vi "acsweep.vi"() -> ()   [LabVIEW 2010]
doc: "I. Description:\nThis example demonstrates how to take a single Measurement (Sample) from an Analog Input Channel.\n\nII. Instructions for Running:\n1. Select the Physical Channel to correspond to where your signal is input on the DAQ device.\n2. Enter the Minimum and Maximum Voltage Ranges\nNote: For better accuracy try to match the Input Ranges to the expected voltage level of the measured signal.\nNote: Use the Gen Voltage Update example to provide a signal on your DAQ device to measure.\n\nIII. Block Diagram Steps:\n1. Create an Analog Input Voltage Channel.\n2. Use the Read VI to Measure 1 Sample from 1 Channel on the Data\nAcquisition Card. Set a timeout so an error is returned if the sample\nis not returned in the specified time limit\n3. Call the Clear Task VI to clear the Task.\n4. Use the popup dialog box to display an error if any.\n\nIV. I/O Connections Overview:\nMake sure your signal input terminal matches the Physical Channel I/O Control."
uses:
  <vilib>/Utility/file.llb/Write To Spreadsheet File (DBL).vi
panel:
  out "Waveform Output":dbl[](graph)
  in  "Physical Channel 2":tag="Dev1/ao0"
  in  "Amplitud":dbl=10.0
  in  "Duracion (s)":dbl=1.0
  in  "stop 2":bool
  out "Waveform Input":dbl[](graph)
  out "Paso #":i32
  in  "Freq Paso":dbl step=0.001 format="%0.3f"
  in  "Freq Hasta":dbl step=0.001 format="%0.3f"
  in  "Freq Desde":dbl step=0.001 format="%0.3f"
  out "Numeric":u32
  in  "Corre":bool
  in  "Maximum Value 2":dbl=10.0 caption="Maximum Value" format="%.2f"
  in  "Minimum Value 2":dbl=-10.0 caption="Minimum Value" format="%0.2f"
  out "In Range?":bool
  in  "stop":bool
  in  "Maximum Value":dbl=10.0 format="%.2f"
  in  "Minimum Value":dbl=-10.0 format="%0.2f"
  in  "Physical Channel":tag="Dev1/ai0"
  # "Channel Parameters"
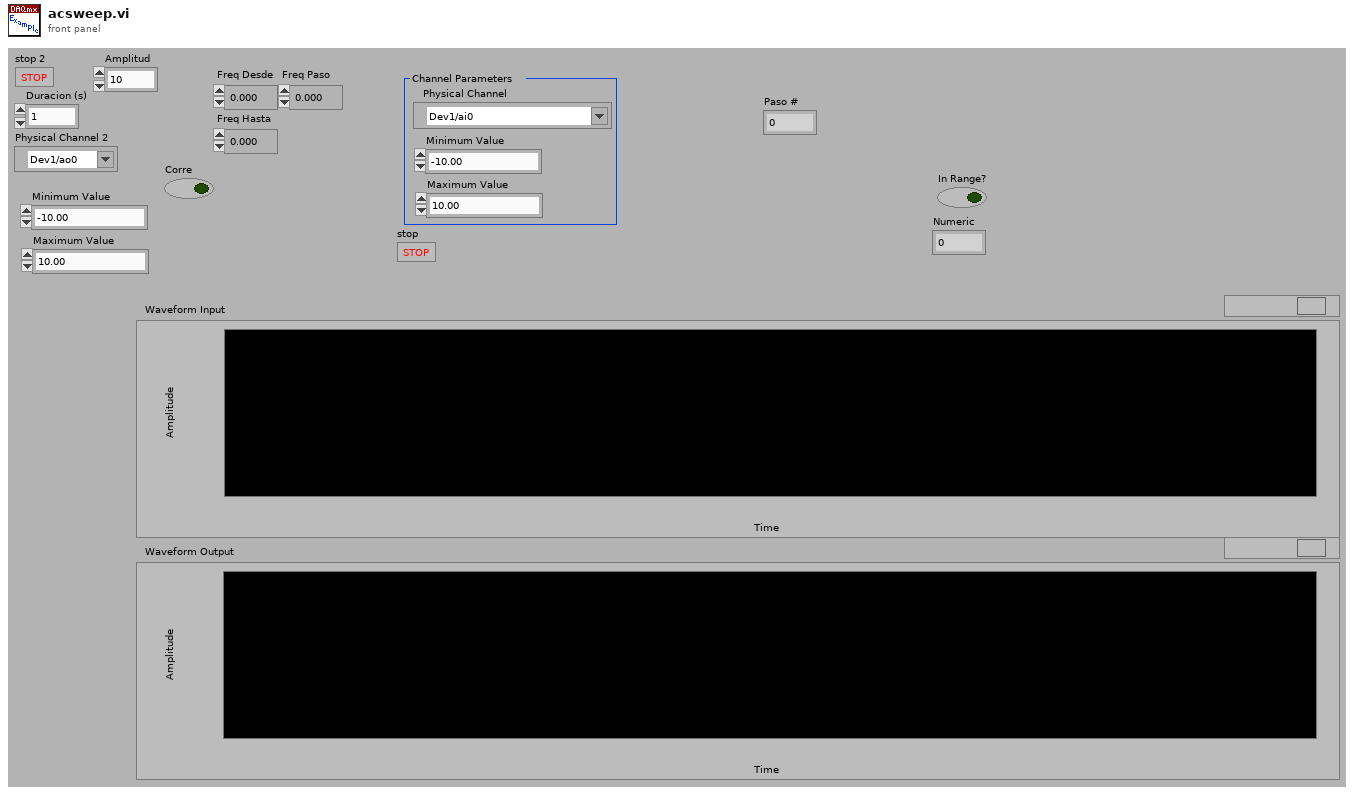
[diagram p1: front panel]
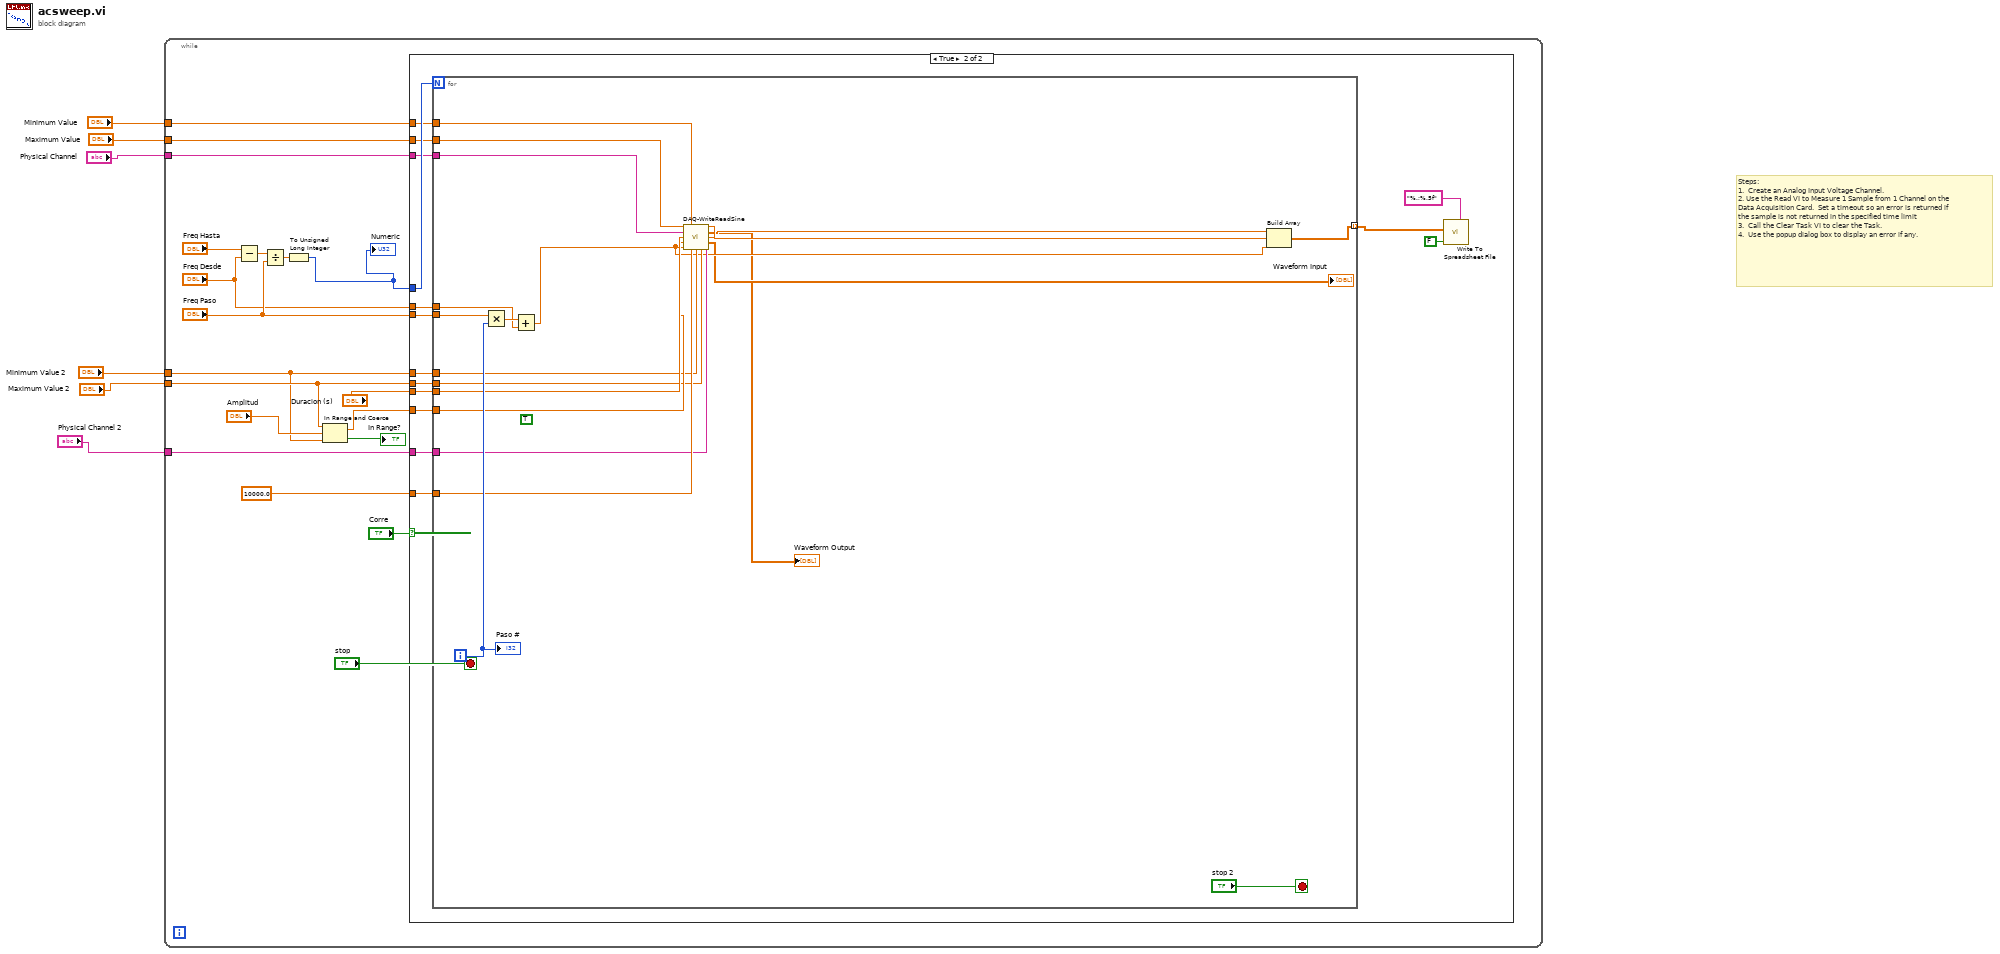
[diagram p0: block diagram]
diagram:
  # "Steps: \n1.  Create an Analog Input Voltage Channel. \n2. Use the Read VI to Measure 1 Sample from 1 Channel on the Data Acquisition Card.  Set a timeout so an error is returned if the sample is not returned in the specified time limit\n3.  Call the Clear Task VI to clear the Task.\n4.  Use the popup dialog box to display an error if any."
  n1 = while {
    tunnel: "Minimum Value" -> [w13]
    tunnel: "Maximum Value" -> [w12]
    tunnel: "Physical Channel" -> [w11]
    tunnel: "Minimum Value 2" -> [w7]
    tunnel: "Maximum Value 2" -> [w8]
    tunnel: "Physical Channel 2" -> [w9]
    stop <- "stop" stop-if-true
    n2 = Subtract(x="Freq Hasta", y="Freq Desde") -> (x-y=w22:dbl)
    n3 = Divide(x=w22, y="Freq Paso") -> (x/y=w21:dbl)
    n4 = To Unsigned Long Integer(number=w21) -> (unsigned 32bit integer=w18:u32)
    "Numeric" <- w18
    n5 = In Range and Coerce(upper limit=w8, x="Amplitud", lower limit=w7) -> (coerced(x)=w15:dbl, In Range?=→"In Range?":bool)
    n6 = case shown="True" "Corre" {
      tunnel: w18 -> [_ w40]
      tunnel: "Freq Paso" -> [_ w39]
      tunnel: "Freq Desde" -> [_ w38]
      tunnel: w15 -> [_ w35]
      tunnel: "Duracion (s)" -> [_ w34]
      tunnel: w13 -> [_ w33]
      tunnel: w12 -> [_ w32]
      tunnel: w11 -> [_ w31]
      tunnel: 10000.0 ("Fs (S/s)") -> [_ w30]
      tunnel: w7 -> [_ w29]
      tunnel: w8 -> [_ w28]
      tunnel: w9 -> [_ w27]
      frame False {
      }
      frame True {
        n7 = for {
          N: w40 -> [_]
          tunnel: w39 -> [w59]
          tunnel: w38 -> [w58]
          tunnel: [w57] -> w26 mode=indexing
          tunnel: w35 -> [w50]
          tunnel: w34 -> [w51]
          tunnel: w33 -> [w54]
          tunnel: w32 -> [w53]
          tunnel: w31 -> [w52]
          tunnel: w30 -> [w49]
          tunnel: w29 -> [w48]
          tunnel: w28 -> [w47]
          tunnel: w27 -> [w46]
          i -> [w56]
          stop <- "stop 2" stop-if-true
          (unwired) TRUE ("auto start")
          n8 = Multiply(x=w59, y=w56) -> (x*y=w60:dbl)
          n9 = Add(x=w60, y=w58) -> (x+y=w43:dbl)
          n10 = call "DAQ-WriteReadSine.vi"("Maximum Input"=w53, "Minimum Input"=w54, "Physical Input Channel"=w52, "tiempo (s)"=w51, "Amplitud"=w50, "Frecuencia"=w43, "Fs (S/s)"=w49, "Minimum Output"=w48, "Maximum Output"=w47, "Physical Output Channel"=w46) -> ("Vout"=w45:dbl, "Output"=→"Waveform Output":dbl[], "Vin"=w44:dbl, "Input"=→"Waveform Input":dbl[])  [unwired: 2 in]
          n11 = Build Array(w44, w45, w43) -> (w57:dbl[])
          "Paso #" <- w56
        }
        n12 = call-poly <vilib>:"Write To Spreadsheet File.vi"("format (%.3f)"="%.;%.5f", "append to file? (new file:F)"=FALSE, "2D data"=w26) -> ()  [unwired: 5 in, 1 out]
      }
    }
  }
